vi "Runout Analizer.vi"(8 "error in":errorcluster, 9 "Variance":dbl min=0.0 max=25.0 step=5.0 format="%.0f %%", 10 "Measurement":i32[](array[numeric]), 11 "Side of first spoke":T3) -> (0 "error out":errorcluster, 2 "Runout Output":T1[](array[typedef]), 3 "Polar Graph":cluster{dbl[], dbl[]}[](graph), 4 "Std Div":dbl, 5 "Min Runout":dbl, 6 "Avg":dbl, 7 "Max Runout":dbl)   [LabVIEW 2025]
uses:
  <vilib>/Analysis/NI_AALBase.lvlib
  Controls/Nippel Turn Direction.ctl
  Controls/Runout Output.ctl
  Controls/Spoke_side.ctl
panel:
  # "Spoke nr 0"
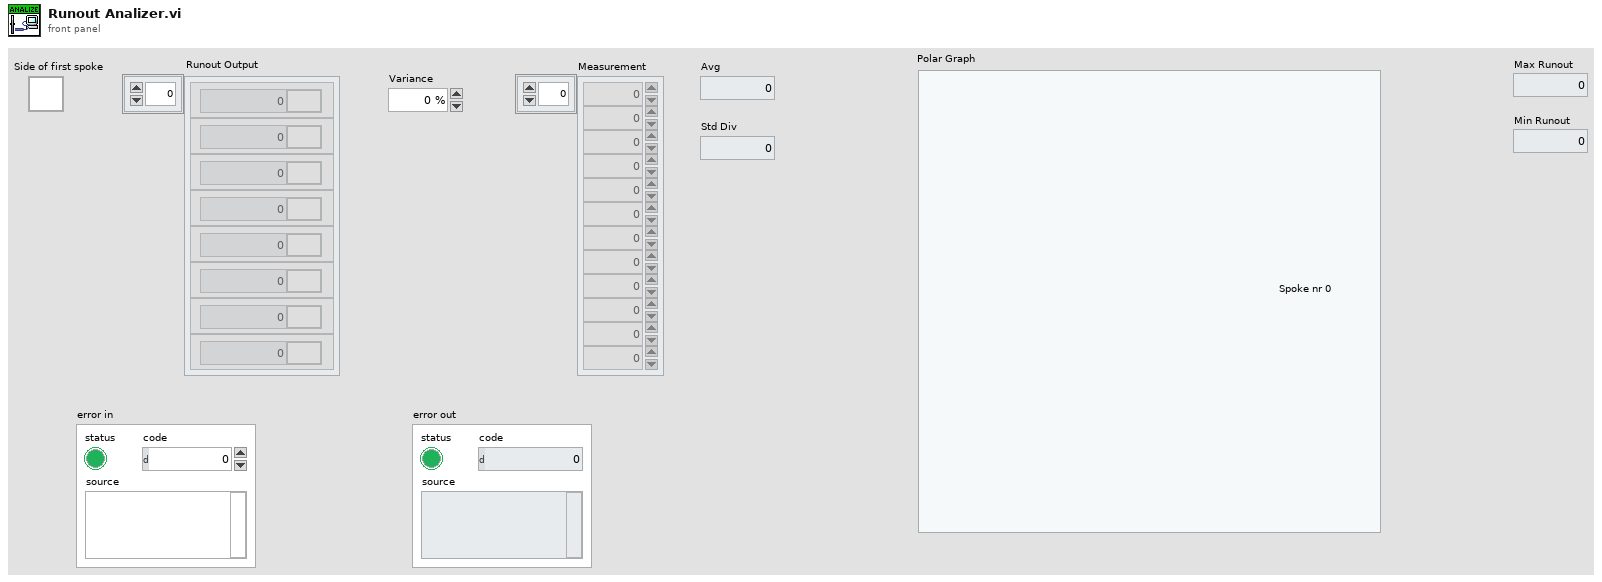
[diagram p1: front panel]
types:
  T1 = typedef "Runout Output.ctl" = cluster{"Value":dbl, "Nippel Direction":T2}
  T2 = typedef "Nippel Turn Direction.ctl" = u16
  T3 = typedef "Spoke_side.ctl" = u16
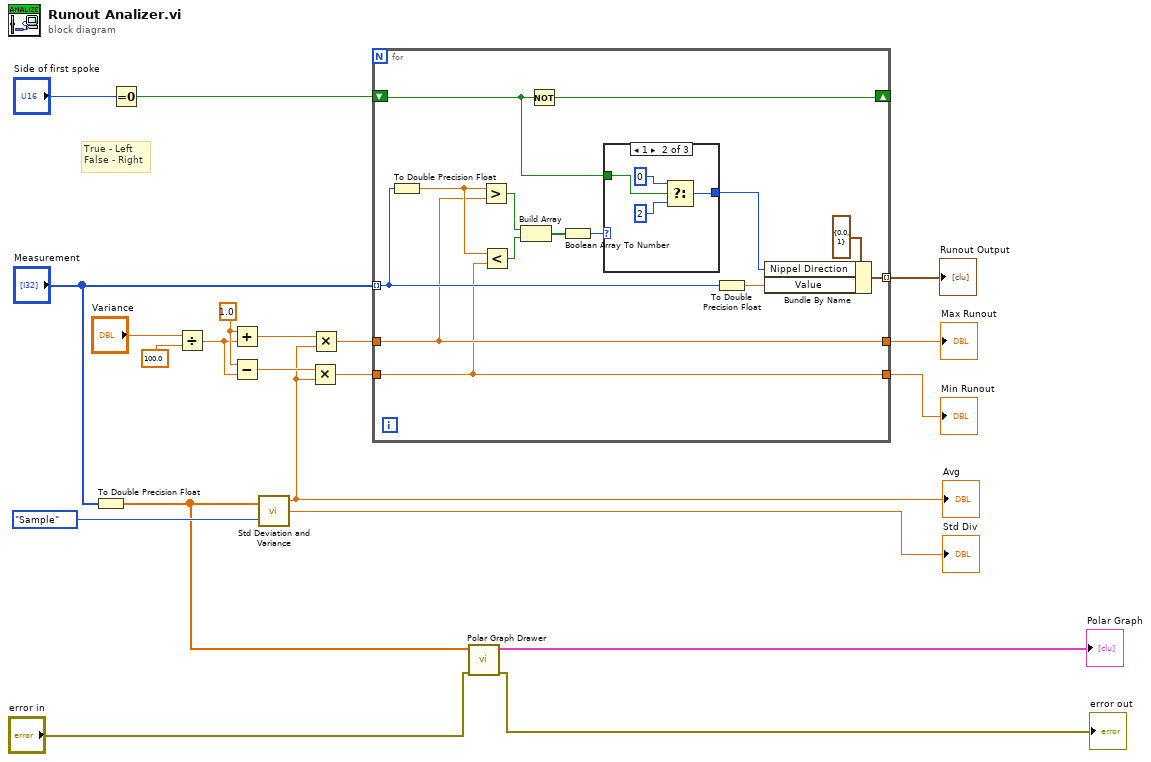
[diagram p0: block diagram]
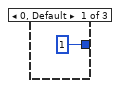
[diagram p2: hidden frame]
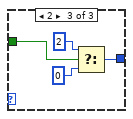
[diagram p3: hidden frame]
diagram:
  w14 = 1.0 ("x")
  # "True - Left\nFalse - Right"
  n1 = To Double Precision Float(number="Measurement") -> (double precision float=w6:dbl[])
  n2 = Equal To 0?(x="Side of first spoke") -> (x = 0?=w20:bool)
  n3 = Divide(x="Variance", y=100.0) -> (x/y=w13:dbl)
  n4 = Add(x=w14, y=w13) -> (x+y=w11:dbl)
  n5 = Subtract(x=w14, y=w13) -> (x-y=w12:dbl)
  n6 = call <vilib>:"Std Deviation and Variance.vi"("X"=w6, "Weighting (Sample)"=enum16{"Sample", "Population"}."Sample") -> ("mean"=w10:dbl, "standard deviation"=→"Std Div":dbl)  [unwired: 1 out]
  "Avg" <- w10
  n7 = Multiply(x=w12, y=w10) -> (x*y=w7:dbl)
  n8 = Multiply(x=w11, y=w10) -> (x*y=w8:dbl)
  n9 = for {
    tunnel: "Measurement" -> [w24] mode=indexing
    tunnel: w8 -> [w23]
    tunnel: w7 -> [w22]
    tunnel: [w35] -> w9 mode=indexing
    shift-right: [w33] -> _
    shift-left: w20 -> [w29]
    tunnel: [w23] -> w2
    tunnel: [w22] -> w1
    n10 = To Double Precision Float(number=w24) -> (double precision float=w31:dbl)
    n11 = Greater?(x=w31, y=w23) -> (0:w25:bool)
    n12 = Less?(x=w31, y=w22) -> (x < y?=w26:bool)
    n13 = Build Array(w25, w26) -> (w30:bool[])
    n14 = Not(x=w29) -> (.not. x?=w33:bool)
    n15 = Boolean Array To Number(Boolean array=w30) -> (number=w27:u32)
    n16 = case shown="1" w27 {
      tunnel: w29 -> [_ w38 w44]
      tunnel: [T2 1 ("Nippel Direction") w37 w41] -> w28
      frame 0, Default {
      }
      frame 1 {
        n17 = Select(t=T2 0 ("Nippel Direction"), s=w38, f=T2 2 ("Nippel Direction")) -> (s? t:f=w37:T2)
      }
      frame 2 {
        n18 = Select(t=T2 2 ("Nippel Direction"), s=w44, f=T2 0 ("Nippel Direction")) -> (s? t:f=w41:T2)
      }
    }
    n19 = To Double Precision Float(number=w24) -> (double precision float=w32:dbl)
    n20 = Bundle By Name(cluster=T1 {"Value"=0.0, "Nippel Direction"=1} ("Runout Output"), "Nippel Direction"=w28, "Value"=w32) -> (w35:T1)
  }
  "Runout Output" <- w9
  "Max Runout" <- w2
  "Min Runout" <- w1
  n21 = call "Polar Graph Drawer.vi"("error in"="error in", "Plot Left"=w6) -> ("error out"=→"error out":errorcluster, "Polar Graph"=→"Polar Graph":cluster{dbl[], dbl[]}[])  [unwired: 8 in]
